vi "Clear_from_Project.vi"(8 "error in (no error)":errorcluster, 11 "Installer in":refnum<class "Installer.lvclass">) -> (0 "error out":errorcluster, 3 "Installer out":refnum<class "Installer.lvclass">)   [LabVIEW 2020, in "Installer.lvclass"]
uses:
  <vilib>/AppBuilder/IB_Classes/Installer/Installer.lvclass
  <vilib>/AppBuilder/IB_Classes/Installer/Installer.lvclass/Installer.ctl
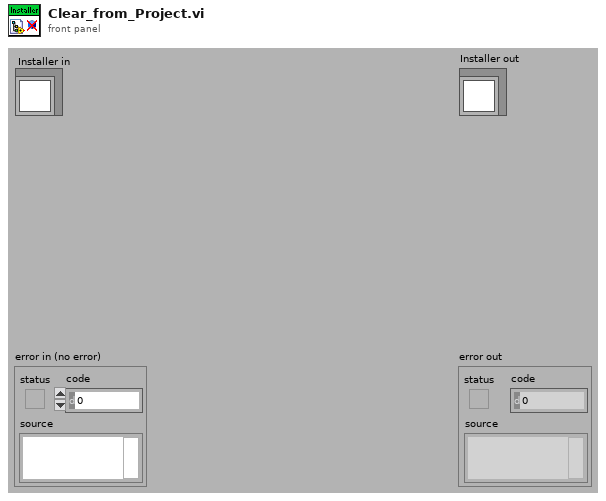
[diagram p1: front panel]
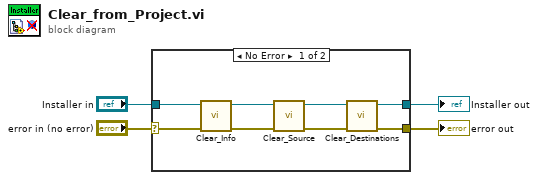
[diagram p0: block diagram]
diagram:
  n1 = case shown="No Error" "error in (no error)" {
    selector: "error in (no error)" -> [w7 w14]
    tunnel: [w5 w14] -> w2
    tunnel: [w6 w13] -> w3
    tunnel: "Installer in" -> [w8 w13]
    frame No Error {
      n2 = call-dynamic "Clear_Info.vi"("error in (no error)"=w7, "Class in"=w8) -> ("error out"=w11:errorcluster, "Class out"=w12:refnum<class "Installer.lvclass">)  [unwired: 8 in]
      n3 = call-dynamic "Clear_Source.vi"("error in (no error)"=w11, "Installer in"=w12) -> ("error out"=w9:errorcluster, "Installer out"=w10:refnum<class "Installer.lvclass">)  [unwired: 8 in]
      n4 = call <vilib>:"Clear_Destinations.vi"("error in (no error)"=w9, "Installer in"=w10) -> ("error out"=w5:errorcluster, "Installer out"=w6:refnum<class "Installer.lvclass">)  [unwired: 8 in]
    }
    frame Error {
    }
  }
  "error out" <- w2
  "Installer out" <- w3
